vi "RunAllTests.vi"() -> ()   [LabVIEW 2019]
uses:
  <vilib>/Rock Robotics/WPI/ThirdParty/JAS_Junk/TrajLib/Trajectory_Library.lvlib
panel:
  out "Meca Drive \nPose Est":bool
  out "Coordinate System":bool
  out "Meca Drive \nOdometry":bool
  out "Meca Drive \nKinematics":bool
  out "Pose3d":bool
  out "Transform3d":bool
  out "Rotation3d":bool
  out "Translation3d":bool
  out "Twist3d":bool
  out "Function Generator \nMatrix":bool
  out "LTV Unicycle \nController":bool
  out "LTV Diff Drive \nController":bool
  out "Time Interpolatable \nRotation2d":bool
  out "Time Interpolatable \nDouble":bool
  out "Time Interpolatable \nBoolean":bool
  out "Time Interpolatable \nPose2d":bool
  out "Implicit Model \nFollower":bool
  out "Function Generator":bool
  out "Diff Drive Accel Limiter":bool
  out "String":string
  out "Vision Utilities":bool
  out "Flywheel Simulation":bool
  out "DC Motor Simulation":bool
  out "Matrix":bool
  out "PID":bool
  out "Profiled PID \nInput/Output":bool
  out "Bang Bang \nInput/Output":bool
  out "Bang Bang Tolerance":bool
  out "Debounce":bool
  out "Math Utils":bool
  out "Linear Filter":bool
  out "State Space Util":bool
  out "Runge Kutta \nTime Varying":bool
  out "Linear System Loop":bool
  out "Swerve Drive \nKinematics":bool
  out "Swerve Drive Odometry":bool
  out "Trajectory Generate":bool
  out "Trajectory Transform":bool
  out "Units":bool
  out "All Tests Finished":bool
  out "Trajectory Concatenate":bool
  out "Trajectory JSON":bool
  out "Diff Drive Train Sim":bool
  out "Timer":bool
  out "Single Jointed \nArm Sim":bool
  out "Elevator Sim":bool
  out "Simple Motor \nFeedforward":bool
  out "Diff Drive Voltage \nConstraint":bool
  out "Diff Drive Pose Est":bool
  out "Holonomic Drive Ctrl":bool
  out "Linear Plant Inv FF":bool
  out "Centrip Accel \nConstraint":bool
  out "Diff Drive Kine \nConstraint":bool
  out "Controller Utility":bool
  out "Swerve Drive Pose Est":bool
  out "Swerve Module State":bool
  out "Trapezoid Profile":bool
  out "Slew Rate Limiter":bool
  out "Chassis Speeds":bool
  out "Numerical Jacobian":bool
  out "Merwe Scaled \nSigma Pts":bool
  out "Numerical Integration":bool
  out "DARE - Ricatti":bool
  out "Quintic Spline":bool
  out "Unscented Kalman \nFilter":bool
  out "Ramsete":bool
  out "Profiled PID":bool
  out "Twist":bool
  out "Translation2d":bool
  out "Transform2d":bool
  out "Rotation2d":bool
  out "Pose2d":bool
  out "Median Filter":bool
  out "Cubic Spline":bool
  out "Linear System ID":bool
  out "Kalman filter":bool
  out "Discretization":bool
  out "PID tolerance":bool
  out "PID Input / Output":bool
  out "Linear Quadradtic \nRegulator":bool
  out "Diff Drive Kinematics":bool
  out "Angle Stats":bool
  # "FORMAL TRAJECTORY / CONTROL LIBRARY TEST PROCEDURE"
  # "FUNCTION NOT\nIMPLEMENTED"
  # "Elipt Region \nConstraint"
  # "Extended Kalman \nFilter"
  # "FUNCTION NOT\nIMPLEMENTED"
  # "Cntrl Affine Plant \nInversion"
  # "FUNCTION NOT\nIMPLEMENTED"
  # "Need to\nimplement test"
  # "Diff Drive Odom"
  # "Rectangular region \nconstraint"
  # "FUNCTION NOT\nIMPLEMENTED"
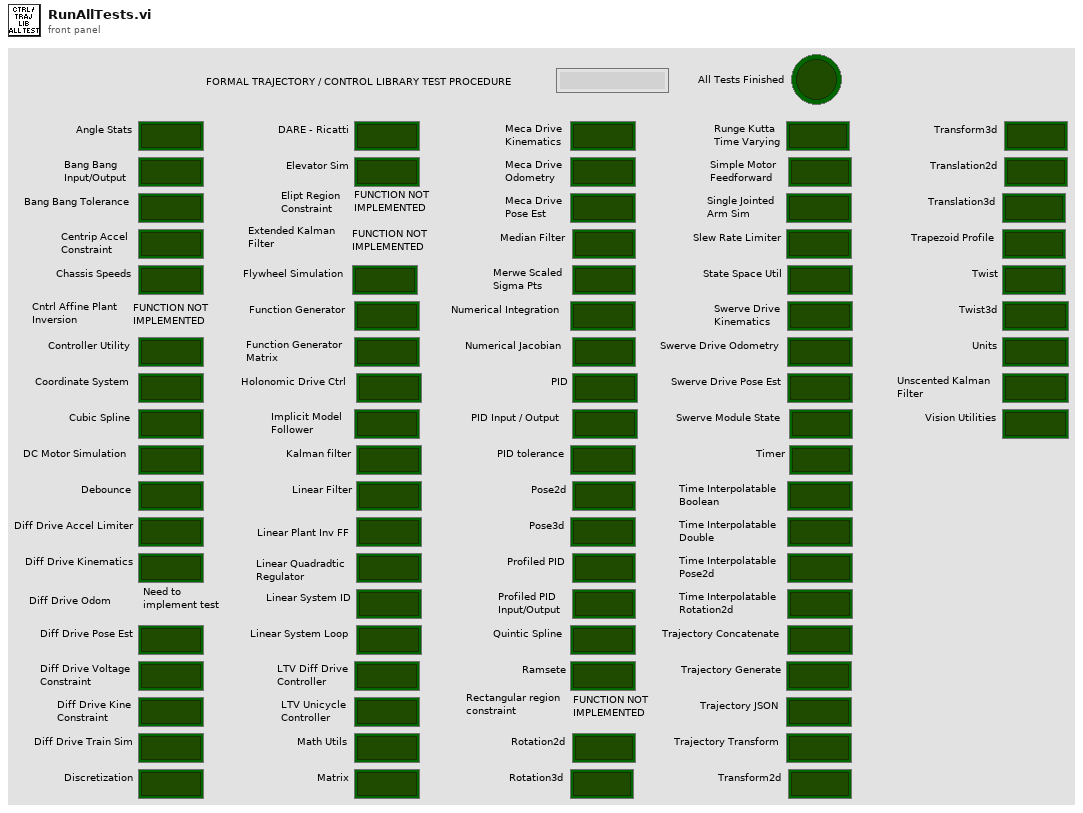
[diagram p1: front panel]
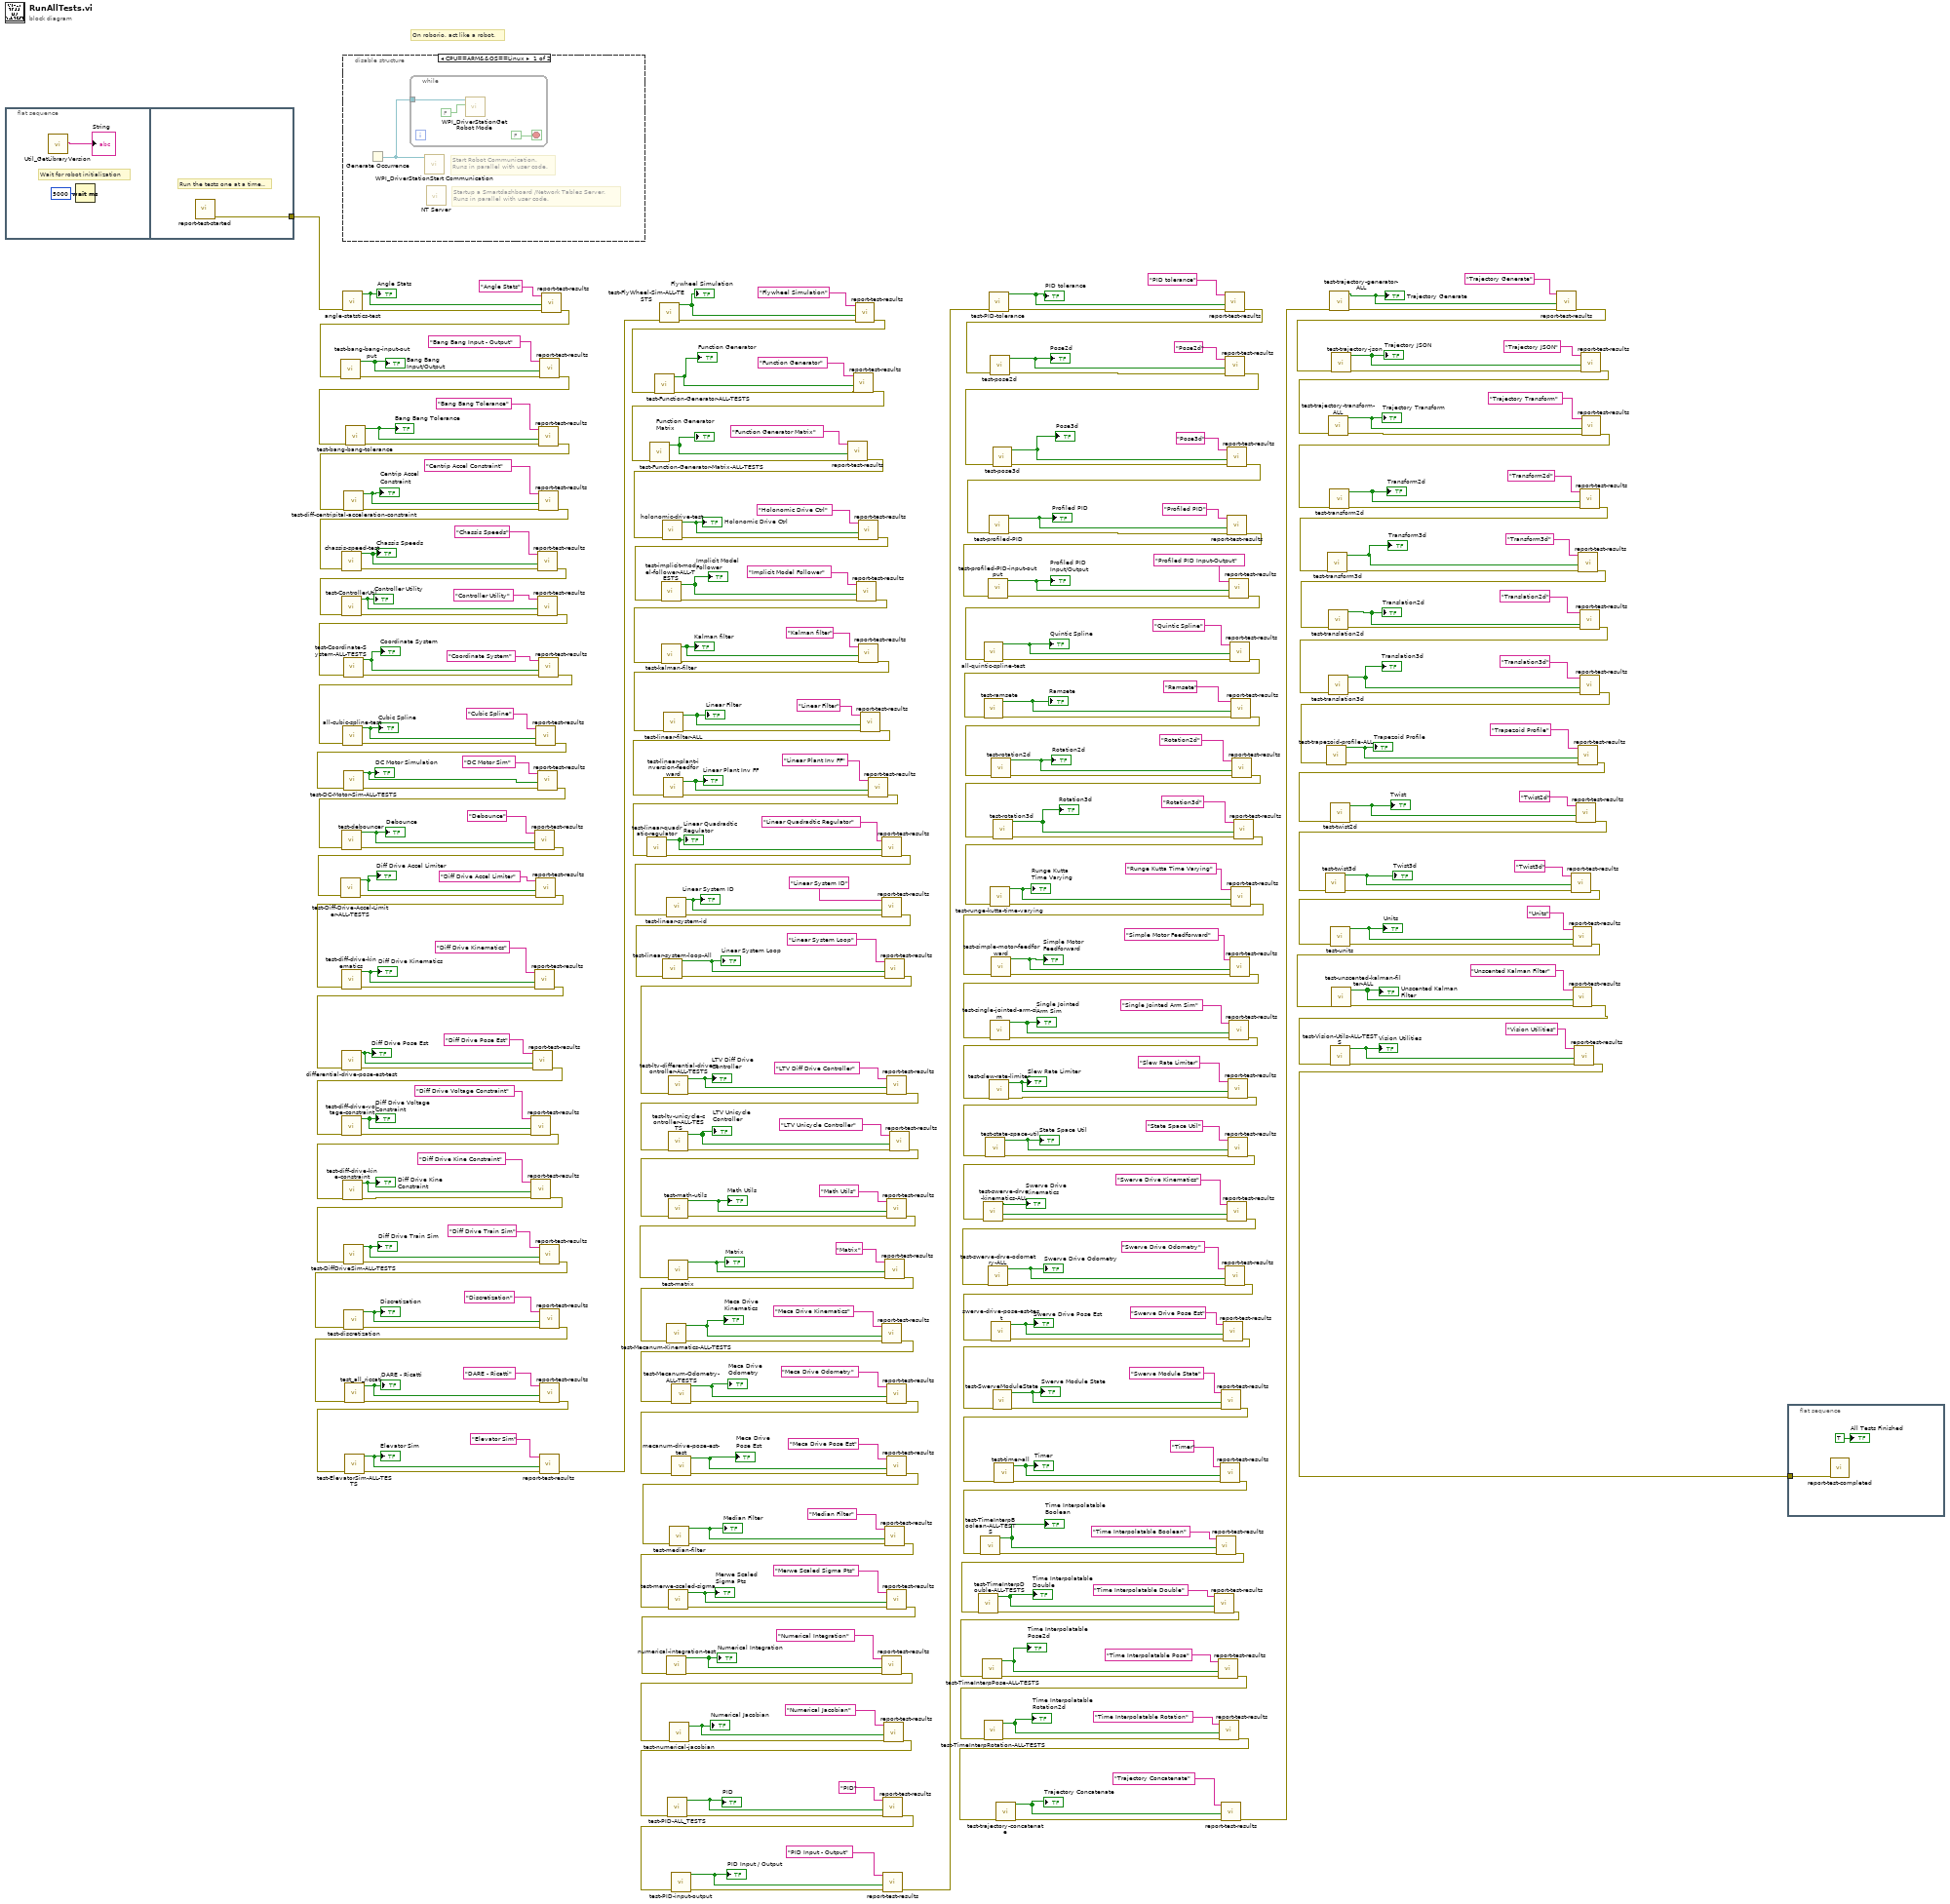
[diagram p0: block diagram]
diagram:
  # "On roborio, act like a robot."
  n1 = flat-sequence {
    tunnel: [w324] -> w104
    frame #0 {
      # "Wait for robot initialization"
      n2 = call <vilib>:"Util_GetLibraryVersion.vi"() -> ("TrajLibVersion"=→"String":string)  [unwired: 11 in]
      n3 = Wait (ms)(milliseconds to wait=u32 5000) -> ()  [unwired: 1 out]
    }
    frame #1 {
      # "Run the tests one at a time.."
      n4 = call "report-test-started.vi"() -> ("error out"=w324:errorcluster)  [unwired: 11 in]
    }
  }
  n5 = disable-structure shown="CPU==ARM&&OS==Linux" {
    frame condition #0 {
      # "Startup a Smartdashboard /Network Tables Server.\nRuns in parallel with user code."
      # "Start Robot Communication.\nRuns in parallel with user code."
      n6 = Generate Occurrence() -> (w325:refnum<k4>)
      n7 = while {
        tunnel: w325 -> [w328]
        stop <- FALSE stop-if-true
        n8 = call <vilib>:"WPI_DriverStationGet Robot Mode.vi"("Finish"=FALSE, "DS Occurrence"=w328) -> ()  [unwired: 10 out]
      }
      n9 = call <vilib>:"WPI_DriverStationStart Communication.vi"("occurrence"=w325) -> ()  [unwired: 2 in, 9 out]
      n10 = call <vilib>:"NT Server.vi"() -> ()  [unwired: 12 in]
    }
    frame condition #1 (active) {
    }
  }
  n11 = call "angle-statstics-test.vi"("error in (no error)"=w104) -> ("error out"=w204:errorcluster, "All Passed"=w321:bool)  [unwired: 9 in]
  "Angle Stats" <- w321
  n12 = call "report-test-results.vi"("error in (no error)"=w204, "TestPassed"=w321, "Test Name"="Angle Stats") -> ("error out"=w205:errorcluster)  [unwired: 8 in]
  n13 = call "test-bang-bang-input-output.vi"("error in (no error)"=w205) -> ("error out"=w203:errorcluster, "All Tests Passed"=w318:bool)  [unwired: 9 in]
  "Bang Bang \nInput/Output" <- w318
  n14 = call "report-test-results.vi"("error in (no error)"=w203, "TestPassed"=w318, "Test Name"="Bang Bang Input - Output") -> ("error out"=w202:errorcluster)  [unwired: 8 in]
  n15 = call "test-bang-bang-tolerance.vi"("error in (no error)"=w202) -> ("error out"=w201:errorcluster, "All Tests Passed"=w316:bool)  [unwired: 9 in]
  "Bang Bang Tolerance" <- w316
  n16 = call "report-test-results.vi"("error in (no error)"=w201, "TestPassed"=w316, "Test Name"="Bang Bang Tolerance") -> ("error out"=w200:errorcluster)  [unwired: 8 in]
  n17 = call "test-diff-centripital-acceleration-constraint.vi"("error in (no error)"=w200) -> ("error out 2"=w199:errorcluster, "Test Passed"=w314:bool)  [unwired: 9 in]
  "Centrip Accel \nConstraint" <- w314
  n18 = call "report-test-results.vi"("error in (no error)"=w199, "TestPassed"=w314, "Test Name"="Centrip Accel Constraint") -> ("error out"=w198:errorcluster)  [unwired: 8 in]
  n19 = call "chassis-speed-test.vi"("error in (no error)"=w198) -> ("error out"=w197:errorcluster, "Test Passed"=w312:bool)  [unwired: 9 in]
  "Chassis Speeds" <- w312
  n20 = call "report-test-results.vi"("error in (no error)"=w197, "TestPassed"=w312, "Test Name"="Chassis Speeds") -> ("error out"=w89:errorcluster)  [unwired: 8 in]
  n21 = call "test-ControllerUtil.vi"("error in (no error)"=w89) -> ("error out"=w196:errorcluster, "All Tests Passed"=w310:bool)  [unwired: 9 in]
  "Controller Utility" <- w310
  n22 = call "report-test-results.vi"("error in (no error)"=w196, "TestPassed"=w310, "Test Name"="Controller Utility") -> ("error out"=w8:errorcluster)  [unwired: 8 in]
  n23 = call "test-Coordinate-System-ALL-TESTS.vi"("error in (no error)"=w8) -> ("error out"=w9:errorcluster, "All Passed"=w6:bool)  [unwired: 9 in]
  "Coordinate System" <- w6
  n24 = call "report-test-results.vi"("error in (no error)"=w9, "TestPassed"=w6, "Test Name"="Coordinate System") -> ("error out"=w7:errorcluster)  [unwired: 8 in]
  n25 = call "all-cubic-spline-test.vi"("error in (no error)"=w7) -> ("error out"=w189:errorcluster, "ALL TESTS PASSED"=w306:bool)  [unwired: 9 in]
  "Cubic Spline" <- w306
  n26 = call "report-test-results.vi"("error in (no error)"=w189, "TestPassed"=w306, "Test Name"="Cubic Spline") -> ("error out"=w103:errorcluster)  [unwired: 8 in]
  n27 = call "test-DC-Motor-Sim-ALL-TESTS.vi"("error in (no error)"=w103) -> ("error out"=w101:errorcluster, "All Passed"=w100:bool)  [unwired: 9 in]
  "DC Motor Simulation" <- w100
  n28 = call "report-test-results.vi"("error in (no error)"=w101, "TestPassed"=w100, "Test Name"="DC Motor Sim") -> ("error out"=w99:errorcluster)  [unwired: 8 in]
  n29 = call "test-debouncer.vi"("error in (no error)"=w99) -> ("error out"=w188:errorcluster, "ALL TESTS PASSED"=w305:bool)  [unwired: 9 in]
  "Debounce" <- w305
  n30 = call "report-test-results.vi"("error in (no error)"=w188, "TestPassed"=w305, "Test Name"="Debounce") -> ("error out"=w86:errorcluster)  [unwired: 8 in]
  n31 = call "test-Diff-Drive-Accel-Limiter-ALL-TESTS.vi"("error in (no error)"=w86) -> ("error out"=w87:errorcluster, "All Passed"=w85:bool)  [unwired: 9 in]
  "Diff Drive Accel Limiter" <- w85
  n32 = call "report-test-results.vi"("error in (no error)"=w87, "TestPassed"=w85, "Test Name"="Diff Drive Accel Limiter") -> ("error out"=w84:errorcluster)  [unwired: 8 in]
  n33 = call "test-diff-drive-kinematics.vi"("error in (no error)"=w84) -> ("error out"=w187:errorcluster, "All Passed"=w304:bool)  [unwired: 9 in]
  "Diff Drive Kinematics" <- w304
  n34 = call "report-test-results.vi"("error in (no error)"=w187, "TestPassed"=w304, "Test Name"="Diff Drive Kinematics") -> ("error out"=w180:errorcluster)  [unwired: 8 in]
  n35 = call "differential-drive-pose-est-test.vi"("error in (no error)"=w180) -> ("error out"=w186:errorcluster, "Test Passed"=w300:bool)  [unwired: 9 in]
  "Diff Drive Pose Est" <- w300
  n36 = call "report-test-results.vi"("error in (no error)"=w186, "TestPassed"=w300, "Test Name"="Diff Drive Pose Est") -> ("error out"=w179:errorcluster)  [unwired: 8 in]
  n37 = call "test-diff-drive-voltage-constraint.vi"("error in (no error)"=w179) -> ("error out 4"=w185:errorcluster, "Test Passed"=w299:bool)  [unwired: 9 in]
  "Diff Drive Voltage \nConstraint" <- w299
  n38 = call "report-test-results.vi"("error in (no error)"=w185, "TestPassed"=w299, "Test Name"="Diff Drive Voltage Constraint") -> ("error out"=w178:errorcluster)  [unwired: 8 in]
  n39 = call "test-diff-drive-kine-constraint.vi"("error in (no error)"=w178) -> ("error out 2"=w184:errorcluster, "Test Passed"=w298:bool)  [unwired: 9 in]
  "Diff Drive Kine \nConstraint" <- w298
  n40 = call "report-test-results.vi"("error in (no error)"=w184, "TestPassed"=w298, "Test Name"="Diff Drive Kine Constraint") -> ("error out"=w177:errorcluster)  [unwired: 8 in]
  n41 = call "test-DiffDriveSim-ALL-TESTS.vi"("error in (no error)"=w177) -> ("error out"=w183:errorcluster, "All Passed"=w294:bool)  [unwired: 9 in]
  "Diff Drive Train Sim" <- w294
  n42 = call "report-test-results.vi"("error in (no error)"=w183, "TestPassed"=w294, "Test Name"="Diff Drive Train Sim") -> ("error out"=w176:errorcluster)  [unwired: 8 in]
  n43 = call "test-discretization.vi"("error in (no error)"=w176) -> ("error out"=w182:errorcluster, "All Tests Passed"=w293:bool)  [unwired: 9 in]
  "Discretization" <- w293
  n44 = call "report-test-results.vi"("error in (no error)"=w182, "TestPassed"=w293, "Test Name"="Discretization") -> ("error out"=w175:errorcluster)  [unwired: 8 in]
  n45 = call "test_all_riccati.vi"("error in (no error)"=w175) -> ("error out"=w181:errorcluster, "All Tests Passed"=w292:bool)  [unwired: 9 in]
  "DARE - Ricatti" <- w292
  n46 = call "report-test-results.vi"("error in (no error)"=w181, "TestPassed"=w292, "Test Name"="DARE - Ricatti") -> ("error out"=w174:errorcluster)  [unwired: 8 in]
  n47 = call "test-ElevatorSim-ALL-TESTS.vi"("error in (no error)"=w174) -> ("error out"=w195:errorcluster, "All Passed"=w288:bool)  [unwired: 9 in]
  "Elevator Sim" <- w288
  n48 = call "report-test-results.vi"("error in (no error)"=w195, "TestPassed"=w288, "Test Name"="Elevator Sim") -> ("error out"=w95:errorcluster)  [unwired: 8 in]
  n49 = call "test-FlyWheel-Sim-ALL-TESTS.vi"("error in (no error)"=w95) -> ("error out"=w97:errorcluster, "All Passed"=w96:bool)  [unwired: 9 in]
  "Flywheel Simulation" <- w96
  n50 = call "report-test-results.vi"("error in (no error)"=w97, "TestPassed"=w96, "Test Name"="Flywheel Simulation") -> ("error out"=w82:errorcluster)  [unwired: 8 in]
  n51 = call "test-Function-Generator-ALL-TESTS.vi"("error in (no error)"=w82) -> ("error out"=w80:errorcluster, "All Passed"=w81:bool)  [unwired: 9 in]
  "Function Generator" <- w81
  n52 = call "report-test-results.vi"("error in (no error)"=w80, "TestPassed"=w81, "Test Name"="Function Generator") -> ("error out"=w45:errorcluster)  [unwired: 8 in]
  n53 = call "test-Function-Generator-Matrix-ALL-TESTS.vi"("error in (no error)"=w45) -> ("error out"=w47:errorcluster, "All Passed"=w46:bool)  [unwired: 9 in]
  "Function Generator \nMatrix" <- w46
  n54 = call "report-test-results.vi"("error in (no error)"=w47, "TestPassed"=w46, "Test Name"="Function Generator Matrix") -> ("error out"=w44:errorcluster)  [unwired: 8 in]
  n55 = call "holonomic-drive-test.vi"("error in (no error)"=w44) -> ("error out"=w194:errorcluster, "ALL TESTS PASSED"=w287:bool)  [unwired: 9 in]
  "Holonomic Drive Ctrl" <- w287
  n56 = call "report-test-results.vi"("error in (no error)"=w194, "TestPassed"=w287, "Test Name"="Holonomic Drive Ctrl") -> ("error out"=w76:errorcluster)  [unwired: 8 in]
  n57 = call "test-implicit-model-follower-ALL-TESTS.vi"("error in (no error)"=w76) -> ("error out"=w78:errorcluster, "All Passed"=w75:bool)  [unwired: 9 in]
  "Implicit Model \nFollower" <- w75
  n58 = call "report-test-results.vi"("error in (no error)"=w78, "TestPassed"=w75, "Test Name"="Implicit Model Follower") -> ("error out"=w77:errorcluster)  [unwired: 8 in]
  n59 = call "test-kalman-filter.vi"("error in (no error)"=w77) -> ("error out"=w193:errorcluster, "ALL TESTS PASSED"=w286:bool)  [unwired: 9 in]
  "Kalman filter" <- w286
  n60 = call "report-test-results.vi"("error in (no error)"=w193, "TestPassed"=w286, "Test Name"="Kalman filter") -> ("error out"=w192:errorcluster)  [unwired: 8 in]
  n61 = call "test-linear-filter-ALL.vi"("error in (no error)"=w192) -> ("error out"=w173:errorcluster, "ALL TESTS GOOD"=w277:bool)  [unwired: 9 in]
  "Linear Filter" <- w277
  n62 = call "report-test-results.vi"("error in (no error)"=w173, "TestPassed"=w277, "Test Name"="Linear Filter") -> ("error out"=w172:errorcluster)  [unwired: 8 in]
  n63 = call "test-linear-plant-inversion-feedforward.vi"("error in (no error)"=w172) -> ("error out"=w171:errorcluster, "All Tests Passed"=w276:bool)  [unwired: 9 in]
  "Linear Plant Inv FF" <- w276
  n64 = call "report-test-results.vi"("error in (no error)"=w171, "TestPassed"=w276, "Test Name"="Linear Plant Inv FF") -> ("error out"=w170:errorcluster)  [unwired: 8 in]
  n65 = call "test-linear-quadratic-regulator.vi"("error in (no error)"=w170) -> ("error out"=w169:errorcluster, "ALL TESTS GOOD"=w275:bool)  [unwired: 9 in]
  "Linear Quadradtic \nRegulator" <- w275
  n66 = call "report-test-results.vi"("error in (no error)"=w169, "TestPassed"=w275, "Test Name"="Linear Quadradtic Regulator") -> ("error out"=w168:errorcluster)  [unwired: 8 in]
  n67 = call "test-linear-system-id.vi"("error in (no error)"=w168) -> ("error out"=w167:errorcluster, "All tests passed"=w274:bool)  [unwired: 9 in]
  "Linear System ID" <- w274
  n68 = call "report-test-results.vi"("error in (no error)"=w167, "TestPassed"=w274, "Test Name"="Linear System ID") -> ("error out"=w159:errorcluster)  [unwired: 8 in]
  n69 = call "test-linear-system-loop-All.vi"("error in (no error)"=w159) -> ("error out"=w160:errorcluster, "ALL TEsts Passed"=w273:bool)  [unwired: 9 in]
  "Linear System Loop" <- w273
  n70 = call "report-test-results.vi"("error in (no error)"=w160, "TestPassed"=w273, "Test Name"="Linear System Loop") -> ("error out"=w53:errorcluster)  [unwired: 8 in]
  n71 = call "test-ltv-differential-drive-controller-ALL-TESTS.vi"("error in (no error)"=w53) -> ("error out"=w54:errorcluster, "All Passed"=w55:bool)  [unwired: 9 in]
  "LTV Diff Drive \nController" <- w55
  n72 = call "report-test-results.vi"("error in (no error)"=w54, "TestPassed"=w55, "Test Name"="LTV Diff Drive Controller") -> ("error out"=w50:errorcluster)  [unwired: 8 in]
  n73 = call "test-ltv-unicycle-controller-ALL-TESTS.vi"("error in (no error)"=w50) -> ("error out"=w52:errorcluster, "All Passed"=w51:bool)  [unwired: 9 in]
  "LTV Unicycle \nController" <- w51
  n74 = call "report-test-results.vi"("error in (no error)"=w52, "TestPassed"=w51, "Test Name"="LTV Unicycle Controller") -> ("error out"=w49:errorcluster)  [unwired: 8 in]
  n75 = call "test-math-utils.vi"("error in (no error)"=w49) -> ("error out"=w158:errorcluster, "ALL TESTS PASSED"=w272:bool)  [unwired: 9 in]
  "Math Utils" <- w272
  n76 = call "report-test-results.vi"("error in (no error)"=w158, "TestPassed"=w272, "Test Name"="Math Utils") -> ("error out"=w157:errorcluster)  [unwired: 8 in]
  n77 = call "test-matrix.vi"("error in (no error)"=w157) -> ("error out"=w161:errorcluster, "All Tests\nPassed"=w271:bool)  [unwired: 9 in]
  "Matrix" <- w271
  n78 = call "report-test-results.vi"("error in (no error)"=w161, "TestPassed"=w271, "Test Name"="Matrix") -> ("error out"=w15:errorcluster)  [unwired: 8 in]
  n79 = call "test-Mecanum-Kinematics-ALL-TESTS.vi"("error in (no error)"=w15) -> ("error out"=w17:errorcluster, "All Passed"=w16:bool)  [unwired: 9 in]
  "Meca Drive \nKinematics" <- w16
  n80 = call "report-test-results.vi"("error in (no error)"=w17, "TestPassed"=w16, "Test Name"="Meca Drive Kinematics") -> ("error out"=w12:errorcluster)  [unwired: 8 in]
  n81 = call "test-Mecanum-Odometry-ALL-TESTS.vi"("error in (no error)"=w12) -> ("error out"=w13:errorcluster, "All Passed"=w11:bool)  [unwired: 9 in]
  "Meca Drive \nOdometry" <- w11
  n82 = call "report-test-results.vi"("error in (no error)"=w13, "TestPassed"=w11, "Test Name"="Meca Drive Odometry") -> ("error out"=w2:errorcluster)  [unwired: 8 in]
  n83 = call "mecanum-drive-pose-est-test.vi"("error in (no error)"=w2) -> ("error out"=w4:errorcluster, "Test Passed"=w3:bool)  [unwired: 9 in]
  "Meca Drive \nPose Est" <- w3
  n84 = call "report-test-results.vi"("error in (no error)"=w4, "TestPassed"=w3, "Test Name"="Meca Drive Pose Est") -> ("error out"=w1:errorcluster)  [unwired: 8 in]
  n85 = call "test-median-filter.vi"("error in (no error)"=w1) -> ("error out"=w162:errorcluster, "ALL TESTS PASSED"=w270:bool)  [unwired: 9 in]
  "Median Filter" <- w270
  n86 = call "report-test-results.vi"("error in (no error)"=w162, "TestPassed"=w270, "Test Name"="Median Filter") -> ("error out"=w156:errorcluster)  [unwired: 8 in]
  n87 = call "test-merwe-scaled-sigma.vi"("error in (no error)"=w156) -> ("error out"=w163:errorcluster, "All Tests Passed"=w256:bool)  [unwired: 9 in]
  "Merwe Scaled \nSigma Pts" <- w256
  n88 = call "report-test-results.vi"("error in (no error)"=w163, "TestPassed"=w256, "Test Name"="Merwe Scaled Sigma Pts") -> ("error out"=w155:errorcluster)  [unwired: 8 in]
  n89 = call "numerical-integration-test.vi"("error in (no error)"=w155) -> ("error out"=w164:errorcluster, "All passed"=w257:bool)  [unwired: 9 in]
  "Numerical Integration" <- w257
  n90 = call "report-test-results.vi"("error in (no error)"=w164, "TestPassed"=w257, "Test Name"="Numerical Integration") -> ("error out"=w154:errorcluster)  [unwired: 8 in]
  n91 = call "test-numerical-jacobian.vi"("error in (no error)"=w154) -> ("error out"=w165:errorcluster, "ALL Tests Passed"=w258:bool)  [unwired: 9 in]
  "Numerical Jacobian" <- w258
  n92 = call "report-test-results.vi"("error in (no error)"=w165, "TestPassed"=w258, "Test Name"="Numerical Jacobian") -> ("error out"=w153:errorcluster)  [unwired: 8 in]
  n93 = call "test-PID-ALL_TESTS.vi"("error in (no error)"=w153) -> ("error out"=w166:errorcluster, "All Passed"=w259:bool)  [unwired: 9 in]
  "PID" <- w259
  n94 = call "report-test-results.vi"("error in (no error)"=w166, "TestPassed"=w259, "Test Name"="PID") -> ("error out"=w152:errorcluster)  [unwired: 8 in]
  n95 = call "test-PID-input-output.vi"("error in (no error)"=w152) -> ("error out"=w190:errorcluster, "All Passed"=w260:bool)  [unwired: 9 in]
  "PID Input / Output" <- w260
  n96 = call "report-test-results.vi"("error in (no error)"=w190, "TestPassed"=w260, "Test Name"="PID Input - Output") -> ("error out"=w191:errorcluster)  [unwired: 8 in]
  n97 = call "test-PID-tolerance.vi"("error in (no error)"=w191) -> ("error out"=w150:errorcluster, "All Tests Passed"=w261:bool)  [unwired: 9 in]
  "PID tolerance" <- w261
  n98 = call "report-test-results.vi"("error in (no error)"=w150, "TestPassed"=w261, "Test Name"="PID tolerance") -> ("error out"=w133:errorcluster)  [unwired: 8 in]
  n99 = call "test-pose2d.vi"("error in (no error)"=w133) -> ("error out"=w149:errorcluster, "All PASSED"=w262:bool)  [unwired: 9 in]
  "Pose2d" <- w262
  n100 = call "report-test-results.vi"("error in (no error)"=w149, "TestPassed"=w262, "Test Name"="Pose2d") -> ("error out"=w21:errorcluster)  [unwired: 8 in]
  n101 = call "test-pose3d.vi"("error in (no error)"=w21) -> ("error out"=w22:errorcluster, "All PASSED"=w19:bool)  [unwired: 9 in]
  "Pose3d" <- w19
  n102 = call "report-test-results.vi"("error in (no error)"=w22, "TestPassed"=w19, "Test Name"="Pose3d") -> ("error out"=w20:errorcluster)  [unwired: 8 in]
  n103 = call "test-profiled-PID.vi"("error in (no error)"=w20) -> ("error out"=w148:errorcluster, "Test Passed 0"=w244:bool)  [unwired: 9 in]
  "Profiled PID" <- w244
  n104 = call "report-test-results.vi"("error in (no error)"=w148, "TestPassed"=w244, "Test Name"="Profiled PID") -> ("error out"=w132:errorcluster)  [unwired: 8 in]
  n105 = call "test-profiled-PID-input-output.vi"("error in (no error)"=w132) -> ("error out"=w147:errorcluster, "All Tests Passed"=w243:bool)  [unwired: 9 in]
  "Profiled PID \nInput/Output" <- w243
  n106 = call "report-test-results.vi"("error in (no error)"=w147, "TestPassed"=w243, "Test Name"="Profiled PID Input-Output") -> ("error out"=w131:errorcluster)  [unwired: 8 in]
  n107 = call "all-quintic-spline-test.vi"("error in (no error)"=w131) -> ("error out"=w146:errorcluster, "ALL TESTS PASSED"=w242:bool)  [unwired: 9 in]
  "Quintic Spline" <- w242
  n108 = call "report-test-results.vi"("error in (no error)"=w146, "TestPassed"=w242, "Test Name"="Quintic Spline") -> ("error out"=w130:errorcluster)  [unwired: 8 in]
  n109 = call "test-ramsete.vi"("error in (no error)"=w130) -> ("error out"=w134:errorcluster, "AtReference End"=w241:bool)  [unwired: 9 in]
  "Ramsete" <- w241
  n110 = call "report-test-results.vi"("error in (no error)"=w134, "TestPassed"=w241, "Test Name"="Ramsete") -> ("error out"=w129:errorcluster)  [unwired: 8 in]
  n111 = call "test-rotation2d.vi"("error in (no error)"=w129) -> ("error out"=w135:errorcluster, "ALL TESTS PASSED"=w240:bool)  [unwired: 9 in]
  "Rotation2d" <- w240
  n112 = call "report-test-results.vi"("error in (no error)"=w135, "TestPassed"=w240, "Test Name"="Rotation2d") -> ("error out"=w31:errorcluster)  [unwired: 8 in]
  n113 = call "test-rotation3d.vi"("error in (no error)"=w31) -> ("error out"=w32:errorcluster, "ALL TESTS PASSED"=w29:bool)  [unwired: 9 in]
  "Rotation3d" <- w29
  n114 = call "report-test-results.vi"("error in (no error)"=w32, "TestPassed"=w29, "Test Name"="Rotation3d") -> ("error out"=w30:errorcluster)  [unwired: 8 in]
  n115 = call "test-runge-kutta-time-varying.vi"("error in (no error)"=w30) -> ("error out"=w136:errorcluster, "Test Passed"=w239:bool)  [unwired: 9 in]
  "Runge Kutta \nTime Varying" <- w239
  n116 = call "report-test-results.vi"("error in (no error)"=w136, "TestPassed"=w239, "Test Name"="Runge Kutta Time Varying") -> ("error out"=w128:errorcluster)  [unwired: 8 in]
  n117 = call "test-simple-motor-feedforward.vi"("error in (no error)"=w128) -> ("error out"=w137:errorcluster, "All Tests Passed"=w238:bool)  [unwired: 9 in]
  "Simple Motor \nFeedforward" <- w238
  n118 = call "report-test-results.vi"("error in (no error)"=w137, "TestPassed"=w238, "Test Name"="Simple Motor Feedforward") -> ("error out"=w127:errorcluster)  [unwired: 8 in]
  n119 = call "test-single-jointed-arm-sim.vi"("error in (no error)"=w127) -> ("error out"=w138:errorcluster, "Test Passed"=w237:bool)  [unwired: 9 in]
  "Single Jointed \nArm Sim" <- w237
  n120 = call "report-test-results.vi"("error in (no error)"=w138, "TestPassed"=w237, "Test Name"="Single Jointed Arm Sim") -> ("error out"=w126:errorcluster)  [unwired: 8 in]
  n121 = call "test-slew-rate-limiter.vi"("error in (no error)"=w126) -> ("error out"=w139:errorcluster, "All Tests Passed"=w236:bool)  [unwired: 9 in]
  "Slew Rate Limiter" <- w236
  n122 = call "report-test-results.vi"("error in (no error)"=w139, "TestPassed"=w236, "Test Name"="Slew Rate Limiter") -> ("error out"=w125:errorcluster)  [unwired: 8 in]
  n123 = call "test-state-space-util.vi"("error in (no error)"=w125) -> ("error out"=w140:errorcluster, "All Tests Passed"=w235:bool)  [unwired: 9 in]
  "State Space Util" <- w235
  n124 = call "report-test-results.vi"("error in (no error)"=w140, "TestPassed"=w235, "Test Name"="State Space Util") -> ("error out"=w124:errorcluster)  [unwired: 8 in]
  n125 = call "test-swerve-drve-kinematics-ALL.vi"("error in (no error)"=w124) -> ("error out"=w141:errorcluster, "ALL TEsts Passed"=w234:bool)  [unwired: 9 in]
  "Swerve Drive \nKinematics" <- w234
  n126 = call "report-test-results.vi"("error in (no error)"=w141, "TestPassed"=w234, "Test Name"="Swerve Drive Kinematics") -> ("error out"=w123:errorcluster)  [unwired: 8 in]
  n127 = call "test-swerve-drve-odometry-ALL.vi"("error in (no error)"=w123) -> ("error out"=w142:errorcluster, "ALL TEsts Passed"=w231:bool)  [unwired: 9 in]
  "Swerve Drive Odometry" <- w231
  n128 = call "report-test-results.vi"("error in (no error)"=w142, "TestPassed"=w231, "Test Name"="Swerve Drive Odometry") -> ("error out"=w122:errorcluster)  [unwired: 8 in]
  n129 = call "swerve-drive-pose-est-test.vi"("error in (no error)"=w122) -> ("error out"=w143:errorcluster, "Test Passed"=w230:bool)  [unwired: 9 in]
  "Swerve Drive Pose Est" <- w230
  n130 = call "report-test-results.vi"("error in (no error)"=w143, "TestPassed"=w230, "Test Name"="Swerve Drive Pose Est") -> ("error out"=w121:errorcluster)  [unwired: 8 in]
  n131 = call "test-SwerveModuleState.vi"("error in (no error)"=w121) -> ("error out"=w144:errorcluster, "ALL TESTS PASSED"=w225:bool)  [unwired: 9 in]
  "Swerve Module State" <- w225
  n132 = call "report-test-results.vi"("error in (no error)"=w144, "TestPassed"=w225, "Test Name"="Swerve Module State") -> ("error out"=w120:errorcluster)  [unwired: 8 in]
  n133 = call "test-timer-all.vi"("error in (no error)"=w120) -> ("error out"=w119:errorcluster, "ALL TESTS PASSED"=w224:bool)  [unwired: 9 in]
  "Timer" <- w224
  n134 = call "report-test-results.vi"("error in (no error)"=w119, "TestPassed"=w224, "Test Name"="Timer") -> ("error out"=w65:errorcluster)  [unwired: 8 in]
  n135 = call "test-TimeInterpBoolean-ALL-TESTS.vi"("error in (no error)"=w65) -> ("error out"=w70:errorcluster, "All Passed"=w67:bool)  [unwired: 9 in]
  "Time Interpolatable \nBoolean" <- w67
  n136 = call "report-test-results.vi"("error in (no error)"=w70, "TestPassed"=w67, "Test Name"="Time Interpolatable Boolean") -> ("error out"=w64:errorcluster)  [unwired: 8 in]
  n137 = call "test-TimeInterpDouble-ALL-TESTS.vi"("error in (no error)"=w64) -> ("error out"=w68:errorcluster, "All Passed"=w66:bool)  [unwired: 9 in]
  "Time Interpolatable \nDouble" <- w66
  n138 = call "report-test-results.vi"("error in (no error)"=w68, "TestPassed"=w66, "Test Name"="Time Interpolatable Double") -> ("error out"=w63:errorcluster)  [unwired: 8 in]
  n139 = call "test-TimeInterpPose-ALL-TESTS.vi"("error in (no error)"=w63) -> ("error out"=w73:errorcluster, "All Passed"=w72:bool)  [unwired: 9 in]
  "Time Interpolatable \nPose2d" <- w72
  n140 = call "report-test-results.vi"("error in (no error)"=w73, "TestPassed"=w72, "Test Name"="Time Interpolatable Pose") -> ("error out"=w60:errorcluster)  [unwired: 8 in]
  n141 = call "test-TimeInterpRotation-ALL-TESTS.vi"("error in (no error)"=w60) -> ("error out"=w61:errorcluster, "All Passed"=w58:bool)  [unwired: 9 in]
  "Time Interpolatable \nRotation2d" <- w58
  n142 = call "report-test-results.vi"("error in (no error)"=w61, "TestPassed"=w58, "Test Name"="Time Interpolatable Rotation") -> ("error out"=w59:errorcluster)  [unwired: 8 in]
  n143 = call "test-trajectory-concatenate.vi"("error in (no error)"=w59) -> ("error out"=w145:errorcluster, "TEsts Passed"=w223:bool)  [unwired: 9 in]
  "Trajectory Concatenate" <- w223
  n144 = call "report-test-results.vi"("error in (no error)"=w145, "TestPassed"=w223, "Test Name"="Trajectory Concatenate") -> ("error out"=w106:errorcluster)  [unwired: 8 in]
  n145 = call "test-trajectory-generator-ALL.vi"("error in (no error)"=w106) -> ("error out"=w151:errorcluster, "ALL TESTS PASSED"=w222:bool)  [unwired: 9 in]
  "Trajectory Generate" <- w222
  n146 = call "report-test-results.vi"("error in (no error)"=w151, "TestPassed"=w222, "Test Name"="Trajectory Generate") -> ("error out"=w105:errorcluster)  [unwired: 8 in]
  n147 = call "test-trajectory-json.vi"("error in (no error)"=w105) -> ("error out 2"=w113:errorcluster, "ALL TESTS PASSED"=w214:bool)  [unwired: 9 in]
  "Trajectory JSON" <- w214
  n148 = call "report-test-results.vi"("error in (no error)"=w113, "TestPassed"=w214, "Test Name"="Trajectory JSON") -> ("error out"=w109:errorcluster)  [unwired: 8 in]
  n149 = call "test-trajectory-transform-ALL.vi"("error in (no error)"=w109) -> ("error out 2"=w112:errorcluster, "Test Passed"=w213:bool)  [unwired: 9 in]
  "Trajectory Transform" <- w213
  n150 = call "report-test-results.vi"("error in (no error)"=w112, "TestPassed"=w213, "Test Name"="Trajectory Transform") -> ("error out"=w108:errorcluster)  [unwired: 8 in]
  n151 = call "test-transform2d.vi"("error in (no error)"=w108) -> ("error out"=w114:errorcluster, "All PASSED"=w212:bool)  [unwired: 9 in]
  "Transform2d" <- w212
  n152 = call "report-test-results.vi"("error in (no error)"=w114, "TestPassed"=w212, "Test Name"="Transform2d") -> ("error out"=w26:errorcluster)  [unwired: 8 in]
  n153 = call "test-transform3d.vi"("error in (no error)"=w26) -> ("error out"=w27:errorcluster, "All PASSED"=w24:bool)  [unwired: 9 in]
  "Transform3d" <- w24
  n154 = call "report-test-results.vi"("error in (no error)"=w27, "TestPassed"=w24, "Test Name"="Transform3d") -> ("error out"=w25:errorcluster)  [unwired: 8 in]
  n155 = call "test-translation2d.vi"("error in (no error)"=w25) -> ("error out"=w115:errorcluster, "All PASSED"=w211:bool)  [unwired: 9 in]
  "Translation2d" <- w211
  n156 = call "report-test-results.vi"("error in (no error)"=w115, "TestPassed"=w211, "Test Name"="Translation2d") -> ("error out"=w35:errorcluster)  [unwired: 8 in]
  n157 = call "test-translation3d.vi"("error in (no error)"=w35) -> ("error out"=w37:errorcluster, "All PASSED"=w36:bool)  [unwired: 9 in]
  "Translation3d" <- w36
  n158 = call "report-test-results.vi"("error in (no error)"=w37, "TestPassed"=w36, "Test Name"="Translation3d") -> ("error out"=w34:errorcluster)  [unwired: 8 in]
  n159 = call "test-trapezoid-profile-ALL.vi"("error in (no error)"=w34) -> ("error out"=w116:errorcluster, "All TEsts passed"=w210:bool)  [unwired: 9 in]
  "Trapezoid Profile" <- w210
  n160 = call "report-test-results.vi"("error in (no error)"=w116, "TestPassed"=w210, "Test Name"="Trapezoid Profile") -> ("error out"=w107:errorcluster)  [unwired: 8 in]
  n161 = call "test-twist2d.vi"("error in (no error)"=w107) -> ("error out"=w117:errorcluster, "All PASSED"=w209:bool)  [unwired: 9 in]
  "Twist" <- w209
  n162 = call "report-test-results.vi"("error in (no error)"=w117, "TestPassed"=w209, "Test Name"="Twist2d") -> ("error out"=w40:errorcluster)  [unwired: 8 in]
  n163 = call "test-twist3d.vi"("error in (no error)"=w40) -> ("error out"=w42:errorcluster, "All PASSED"=w41:bool)  [unwired: 9 in]
  "Twist3d" <- w41
  n164 = call "report-test-results.vi"("error in (no error)"=w42, "TestPassed"=w41, "Test Name"="Twist3d") -> ("error out"=w39:errorcluster)  [unwired: 8 in]
  n165 = call "test-units.vi"("error in (no error)"=w39) -> ("error out"=w111:errorcluster, "All Tests Passed"=w208:bool)  [unwired: 9 in]
  "Units" <- w208
  n166 = call "report-test-results.vi"("error in (no error)"=w111, "TestPassed"=w208, "Test Name"="Units") -> ("error out"=w110:errorcluster)  [unwired: 8 in]
  n167 = call "test-unscented-kalman-filter-ALL.vi"("error in (no error)"=w110) -> ("error out"=w118:errorcluster, "All Tests Passed"=w206:bool)  [unwired: 9 in]
  "Unscented Kalman \nFilter" <- w206
  n168 = call "report-test-results.vi"("error in (no error)"=w118, "TestPassed"=w206, "Test Name"="Unscented Kalman Filter") -> ("error out"=w93:errorcluster)  [unwired: 8 in]
  n169 = call "test-Vision-Utils-ALL-TESTS.vi"("error in (no error)"=w93) -> ("error out"=w92:errorcluster, "All Passed"=w91:bool)  [unwired: 9 in]
  "Vision Utilities" <- w91
  n170 = call "report-test-results.vi"("error in (no error)"=w92, "TestPassed"=w91, "Test Name"="Vision Utilities") -> ("error out"=w90:errorcluster)  [unwired: 8 in]
  n171 = flat-sequence {
    tunnel: w90 -> [w329]
    frame #0 {
      n172 = call "report-test-completed.vi"("error in (no error)"=w329) -> ()  [unwired: 10 in, 1 out]
      "All Tests Finished" <- TRUE ("All Tests Finished")
    }
  }
